vi "Prova filtraggio.vi"() -> ()   [LabVIEW 2019]
uses:
  <vilib>/DAQmx/read.llb/DAQmx Read (Analog Wfm 1Chan NSamp).vi
  <vilib>/DAQmx/create/channels.llb/DAQmx Create Channel (AI-Voltage-Basic).vi
  <vilib>/DAQmx/configure/timing.llb/DAQmx Timing (Sample Clock).vi
  <vilib>/DAQmx/miscellaneous.llb/DAQmx Fill In Error Info.vi
  <vilib>/express/express analysis/Spectral/Block/exnSpectralBlock spectral measurements peak poly.vi
  <vilib>/express/express analysis/Spectral/Block/exnSpectralBlock spectral measurements peak WFM.vi
  <vilib>/express/express analysis/Spectral/XNode/ExpressSpectralMeasurementsBlockNode.xnode
panel:
  out "Waveform Chart":waveform(dbl)(graph)
  out "loop Iteration":i32
  out "Waveform Graph":cluster{"f0":dbl, "df":dbl, "magnitude":dbl[]}(graph)
  in  "rate":dbl=20000.0 format="%0.2f"
  in  "sample mode":i32(ring)=10123 items=["Finite Samples"=10178, "Continuous Samples"=10123, "Hardware Timed Single Point"=12522]
  in  "samples per channel":i32=200000
  in  "stop":bool
  in  "MODULE NAME":string="cDAQ9181-1B4068CMod1"
  in  "error in":errorcluster
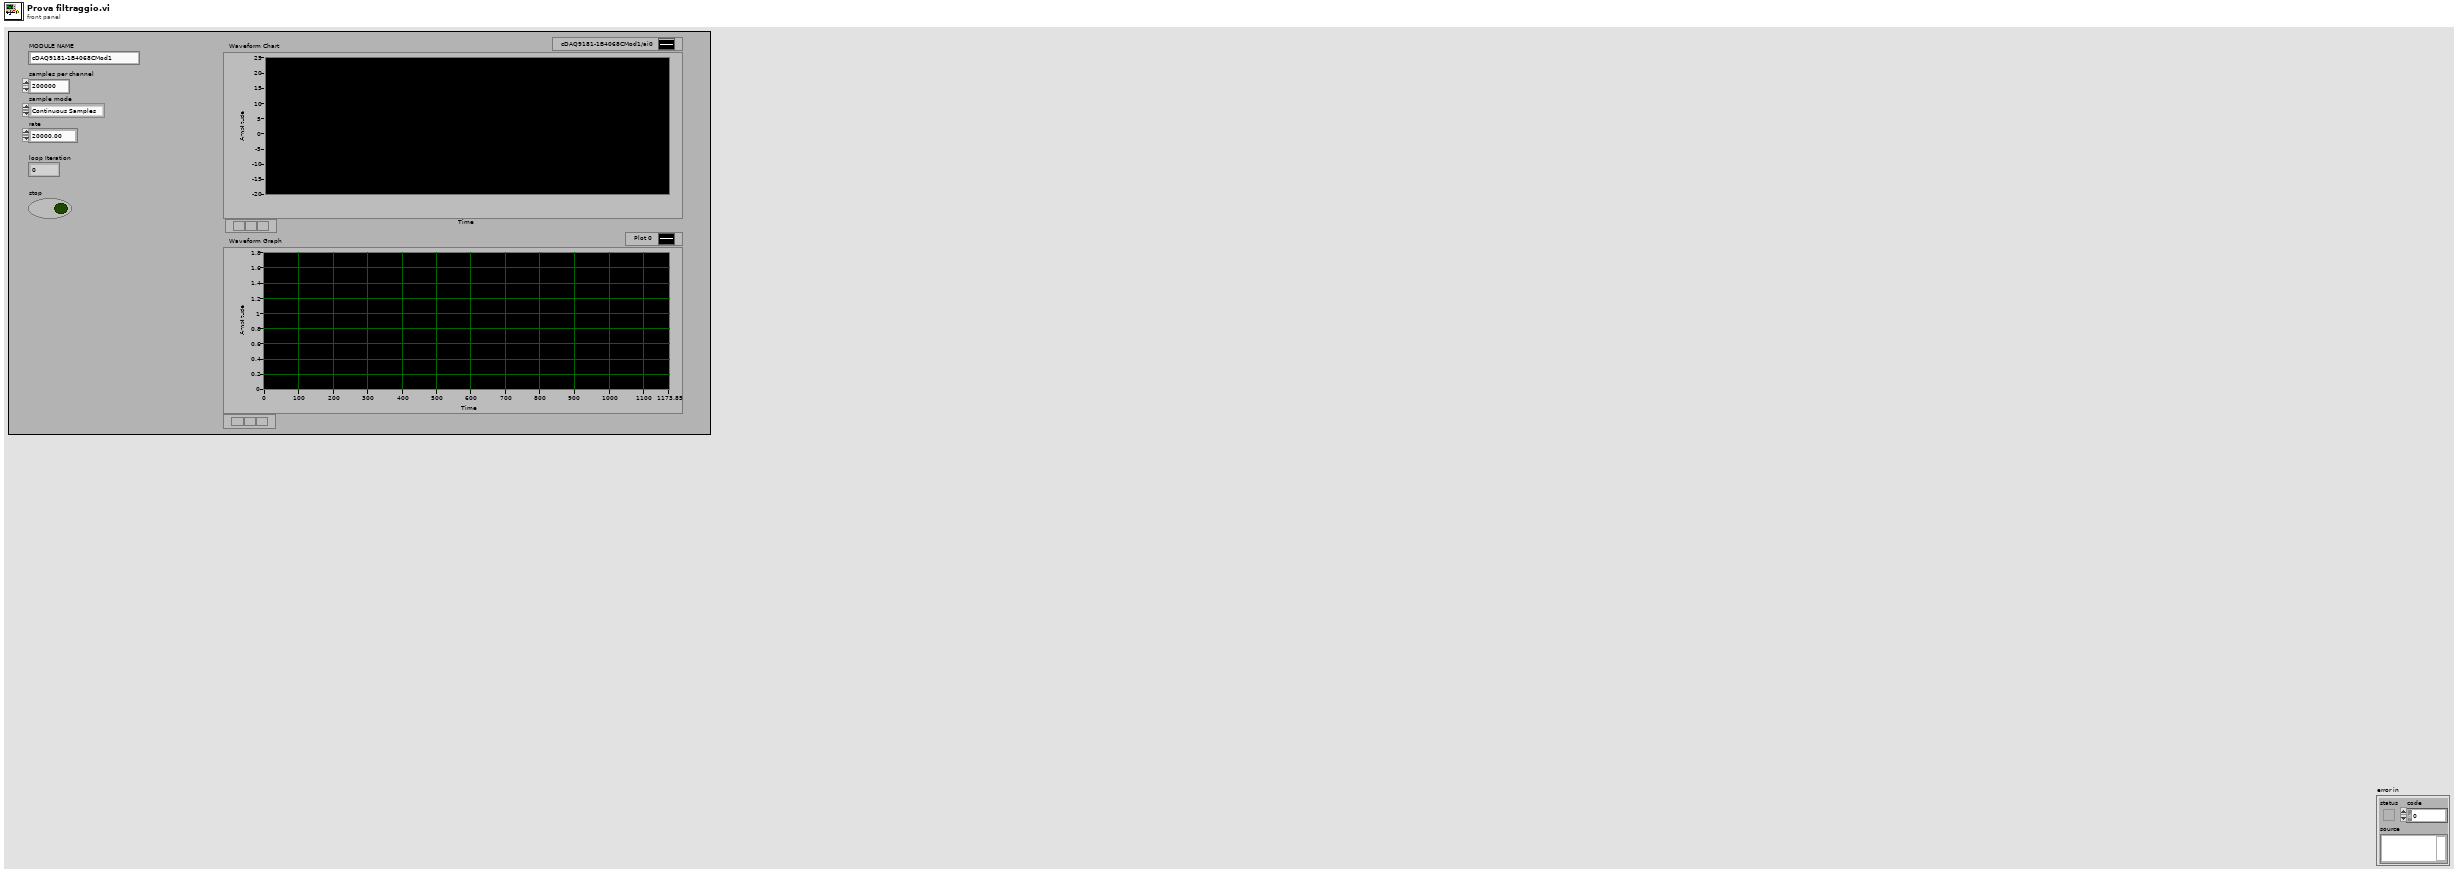
[diagram p1: front panel]
types:
  T1 = cluster{"averaging mode":u16, "weighting mode":u16, "number of averages":u32}
  T2 = cluster{"dB On (F)":bool, "unwrap phase (F)":bool, "convert to degree (F)":bool}
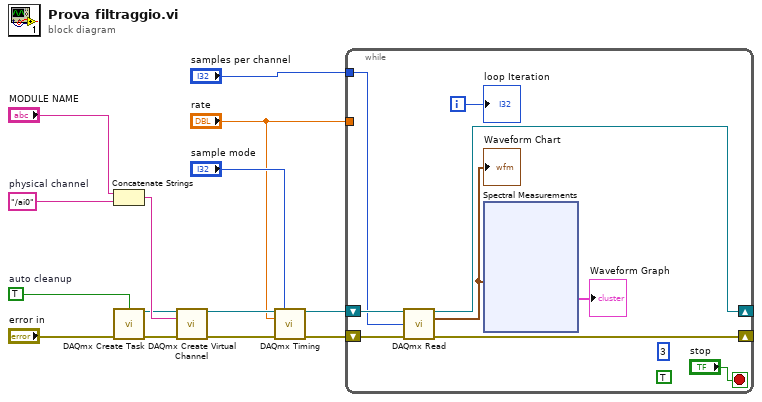
[diagram p0: block diagram]
diagram:
  w13 = "/ai0"  # physical channel
  w11 = TRUE  # auto cleanup
  n1 = Concatenate Strings("MODULE NAME", w13) -> (w14:string)
  n2 = call <vilib>:"DAQmx Create Task.vi"("auto cleanup"=w11, "error in"="error in") -> ("task out"=w12:refnum<k21>, "error out"=w10:errorcluster)  [unwired: 12 in]
  n3 = call-poly <vilib>:"DAQmx Create Virtual Channel.vi"("task in"=w12, "physical channels"=w14, "error in"=w10) -> ("task out"=w7:refnum<k21>, "error out"=w6:errorcluster)  [unwired: 11 in]
  n4 = call-poly <vilib>:"DAQmx Timing.vi"("task/channels in"=w7, "sample mode"="sample mode", "rate"="rate", "error in"=w6) -> ("task out"=w5:refnum<k21>, "error out"=w4:errorcluster)  [unwired: 10 in]
  n5 = while {
    shift-right: [w23] -> _
    shift-left: w5 -> [w18]
    shift-right: [w21] -> _
    shift-left: w4 -> [w22]
    tunnel: "rate" -> [_]
    tunnel: "samples per channel" -> [w16]
    i -> [w17]
    stop <- "stop" stop-if-true
    (unwired) 3 ("order")
    (unwired) TRUE ("init/cont (init:F)")
    n6 = call-poly <vilib>:"DAQmx Read.vi"("task/channels in"=w18, "number of samples per channel"=w16, "error in"=w22) -> ("task out"=w23:refnum<k21>, "data"=w15:waveform(dbl), "error out"=w21:errorcluster)  [unwired: 10 in]
    "Waveform Chart" <- w15
    n7 = xnode "Spectral Measurements"("Signals"=w15) -> ("FFT - (Peak)"=→"Waveform Graph":cluster{"f0":dbl, "df":dbl, "magnitude":dbl[]})  [unwired: 1 in, 2 out]
    "loop Iteration" <- w17
  }
